vi "Fetch (U64 Array).vi"(6 "default timestamp":timestamp, 7 "PV name":string, 8 "error in":errorcluster, 10 "default value":u64[](array[numeric]), 11 "Server in":refnum<class "Server.lvclass">) -> (0 "error out":errorcluster, 1 "PV not found?":bool, 2 "value":u64[](array[numeric]), 3 "Server out":refnum<class "Server.lvclass">, 4 "timestamp":timestamp)   [LabVIEW 2020, in "PV Access.lvlib" / "PVA Server.lvlib" / "Server.lvclass"]
uses:
  Server.lvclass
  PV Data/PV Data/PV Data.lvclass
  Source/Source.lvclass
  Server.lvclass/Server.ctl
  72f90cc3-0893-4152-b792-4968517a4130.vi
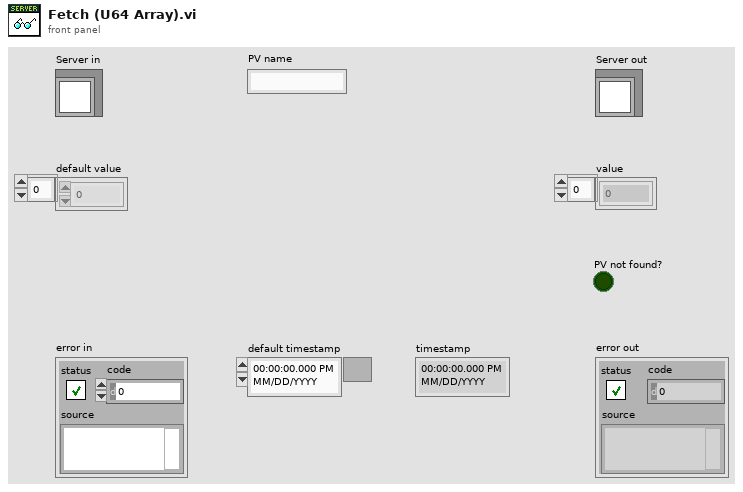
[diagram p1: front panel]
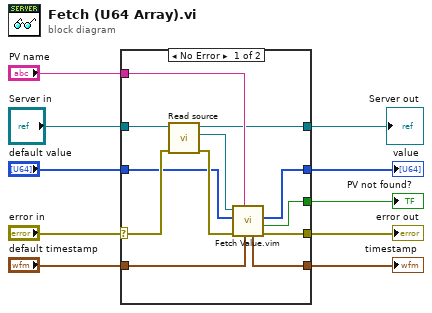
[diagram p0: block diagram]
diagram:
  n1 = case shown="No Error" "error in" {
    selector: "error in" -> [w20 w24]
    tunnel: [w22 w24] -> w10
    tunnel: "PV name" -> [w21 _]
    tunnel: [w19 w23] -> w7
    tunnel: "Server in" -> [w17 w26]
    tunnel: [w16 w26] -> w5
    tunnel: "default value" -> [w14 w25]
    tunnel: [w13 w25] -> w3
    tunnel: "default timestamp" -> [w12 w23]
    tunnel: [w11 _] -> w1
    frame No Error {
      n2 = call "Read source.vi"("error in (no error)"=w20, "Server in"=w17) -> ("error out"=w18:errorcluster, "Source"=w15:refnum<class "Source.lvclass">, "Server out"=w16:refnum<class "Server.lvclass">)  [unwired: 7 in]
      n3 = call "Fetch Value.vim"("default timestamp"=w12, "PV name"=w21, "error in"=w18, "default value"=w14, "Source in"=w15) -> ("error out"=w22:errorcluster, "PV not found?"=w11:bool, "value"=w13:u64[], "timestamp"=w19:timestamp)  [unwired: 2 in, 1 out]
    }
    frame Error {
    }
  }
  "Server out" <- w5
  "error out" <- w10
  "timestamp" <- w7
  "value" <- w3
  "PV not found?" <- w1
